vi "Init WS Manager.vi"(8 "error in (no error)":errorcluster, 11 "Basic WebSocket Manager in":refnum<class "Basic WebSocket Manager.lvclass">) -> (0 "error out":errorcluster, 3 "Basic WebSocket Manager out":refnum<class "Basic WebSocket Manager.lvclass">)   [LabVIEW 2020, in "HTTP Server.lvlib" / "Basic WebSocket Manager.lvclass"]
uses:
  Basic WebSocket Manager.lvclass
  Basic WebSocket Manager.lvclass/Basic WebSocket Manager.ctl
  WebSocket Client/WebSocket Client.lvclass
  Ref Data.ctl
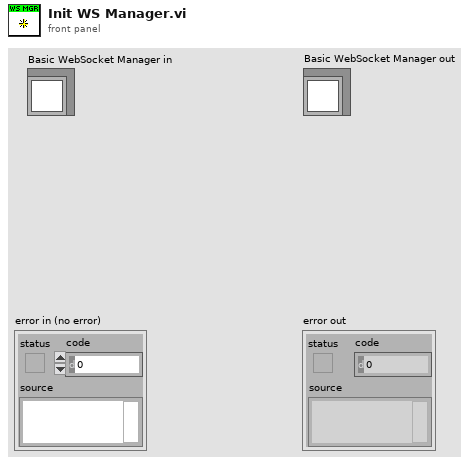
[diagram p1: front panel]
types:
  T1 = typedef "HTTP Server.lvlib/Basic WebSocket Manager.lvclass/Ref Data.ctl" = cluster{"Clients":map{string, refnum<class "WebSocket Client.lvclass">}}
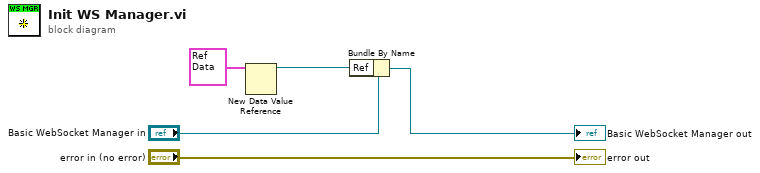
[diagram p0: block diagram]
diagram:
  n1 = New Data Value Reference(data value=T1 {"Clients"={}} ("Ref Data")) -> (data value reference=w1:refnum<data-value>)  [unwired: 1 in, 1 out]
  n2 = Bundle By Name(cluster="Basic WebSocket Manager in", "Ref"=w1) -> (→"Basic WebSocket Manager out":refnum<class "Basic WebSocket Manager.lvclass">)
  "error out" <- "error in (no error)"
